vi "RunVIAnalyzer.vi"() -> ()   [LabVIEW 2020]
uses:
  <vilib>/addons/analyzer/_analyzerctrls.llb/VIAnCtl Results.ctl
  <vilib>/addons/analyzer/_analyzerctrls.llb/VIAnCtl ResultsData (index).ctl
  <vilib>/addons/analyzer/_analyzerctrls.llb/VIAnCtl ResultStatus.ctl
  <vilib>/addons/analyzer/_vianresshared.llb/VIAnRes Parsed Results Data (by VI).ctl
  <vilib>/addons/analyzer/_vianresshared.llb/VIAnRes Parsed Results Data (by Test).ctl
  <vilib>/addons/analyzer/_analyzerctrls.llb/VIAnCtl Test Config Data.ctl
  <vilib>/addons/analyzer/_analyzerctrls.llb/VIAnCtl TestRanking.ctl
  <vilib>/addons/analyzer/_analyzerctrls.llb/VIAnCtl Config Control Value.ctl
  <vilib>/Wiresmith Technology/G CLI/CLI Class/CLI.lvclass
  <vilib>/addons/analyzer/NI_VIAnalyzerTKVIs.lvlib
panel:
  out "Analysis Results":T9 {"Test Config Data"."Test Ranking" items=["Low", "Normal", "High"]}
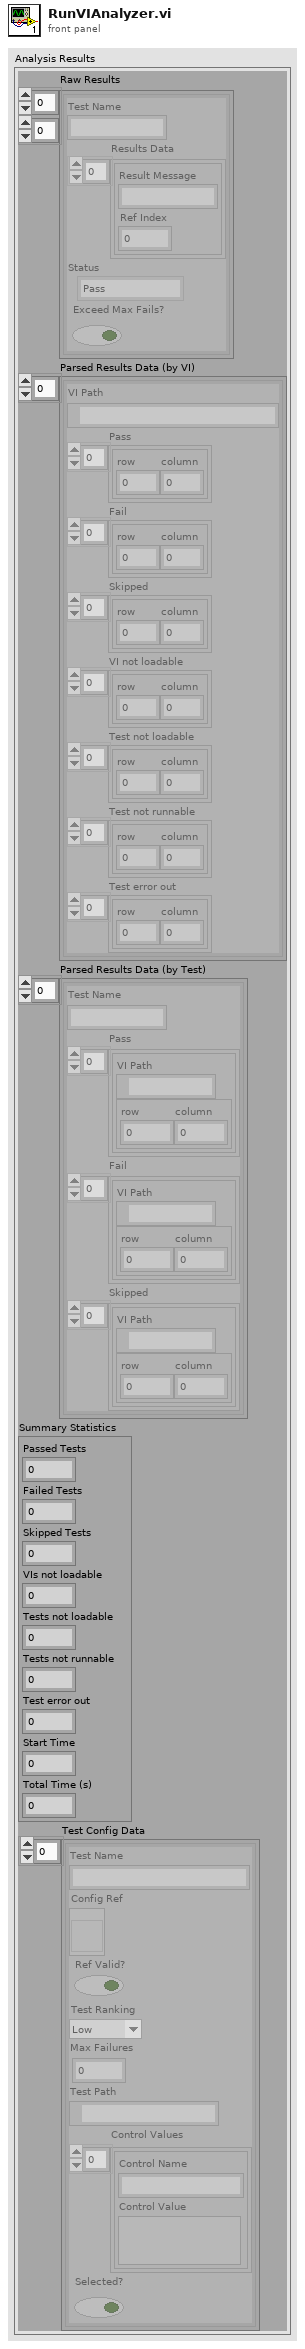
[diagram p1: front panel]
types:
  T1 = typedef "VIAnCtl Results.ctl" = cluster{"Test Name":string, "Results Data":T2[], "Status":T3, "Exceed Max Fails?":bool}
  T2 = typedef "VIAnCtl ResultsData (index).ctl" = cluster{"Result Message":string, "Ref Index":i32}
  T3 = typedef "VIAnCtl ResultStatus.ctl" = enum16{"Pass", "Fail", "Skipped", "VI not loadable", "Test not loadable", "Test not runnable", "Test error out"}
  T4 = typedef "VIAnRes Parsed Results Data (by VI).ctl" = cluster{"VI Path":path, "Pass":cluster{"row":i32, "column":i32}[], "Fail":cluster{"row":i32, "column":i32}[], "Skipped":cluster{"row":i32, "column":i32}[], "VI not loadable":cluster{"row":i32, "column":i32}[], "Test not loadable":cluster{"row":i32, "column":i32}[], "Test not runnable":cluster{"row":i32, "column":i32}[], "Test error out":cluster{"row":i32, "column":i32}[]}
  T5 = typedef "VIAnRes Parsed Results Data (by Test).ctl" = cluster{"Test Name":string, "Pass":cluster{"VI Path":path, "index":cluster{"row":i32, "column":i32}}[], "Fail":cluster{"VI Path":path, "index":cluster{"row":i32, "column":i32}}[], "Skipped":cluster{"VI Path":path, "index":cluster{"row":i32, "column":i32}}[]}
  T6 = typedef "VIAnCtl Test Config Data.ctl" = cluster{"Test Name":string, "Config Ref":refnum<vi>, "Ref Valid?":bool, "Test Ranking":T7, "Max Failures":u32, "Test Path":path, "Control Values":T8[], "Selected?":bool}
  T7 = typedef "VIAnCtl TestRanking.ctl" = u16
  T8 = typedef "VIAnCtl Config Control Value.ctl" = cluster{"Control Name":string, "Control Value":variant}
  T9 = cluster{"Raw Results":T1[][], "Parsed Results Data (by VI)":T4[], "Parsed Results Data (by Test)":T5[], "Summary Statistics":cluster{"Passed Tests":i32, "Failed Tests":i32, "Skipped Tests":i32, "VIs not loadable":i32, "Tests not loadable":i32, "Tests not runnable":i32, "Test error out":i32, "Start Time":u32, "Total Time (s)":dbl}, "Test Config Data":T6[]}
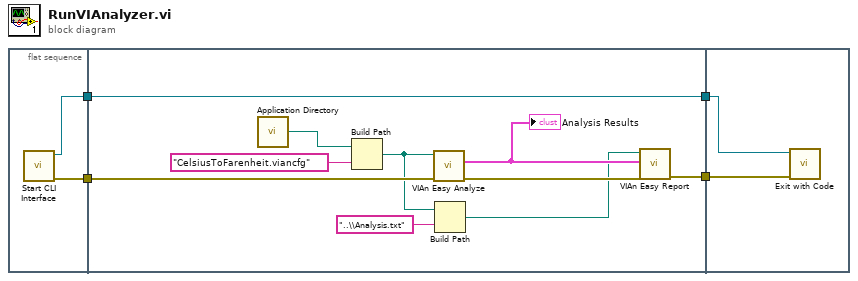
[diagram p0: block diagram]
diagram:
  n1 = flat-sequence {
    tunnel: [w6] -> w4
    tunnel: [w5] -> w1
    tunnel: w4 -> [w10]
    tunnel: [w15] -> w3
    tunnel: [w13] -> w2
    tunnel: w1 -> [w13]
    tunnel: w3 -> [w18]
    tunnel: w2 -> [w17]
    frame #0 {
      n2 = call <vilib>:"Start CLI Interface.vi"() -> ("error out"=w6:errorcluster, "CLI out"=w5:refnum<class "CLI.lvclass">)  [unwired: 8 in, 2 out]
    }
    frame #1 {
      n3 = call <vilib>:"Application Directory.vi"() -> ("Application Directory"=w9:path)
      n4 = Build Path(base path=w9, name or relative path="CelsiusToFarenheit.viancfg") -> (appended path=w7:path)
      n5 = call <vilib>:"VIAn Easy Analyze.vi"("error in (no error)"=w10, "Analysis Target"=w7) -> ("error out"=w16:errorcluster, "Analysis Results"=w14:T9)  [unwired: 8 in]
      "Analysis Results" <- w14
      n6 = Build Path(base path=w7, name or relative path="..\\Analysis.txt") -> (appended path=w11:path)
      n7 = call <vilib>:"VIAn Easy Report.vi"("error in (no error)"=w16, "Analysis Results"=w14, "Report Save Path"=w11) -> ("error out"=w15:errorcluster)  [unwired: 8 in]
    }
    frame #2 {
      n8 = call <vilib>:"Exit with Code.vi"("error in (no error)"=w18, "CLI in"=w17) -> ()  [unwired: 9 in, 1 out]
    }
  }
